vi "FlatToRichcif_channelcore_ForceChannel.vi"(5 "OutputClusterType":T1, 11 "InputCluster":T2) -> (3 "OutputCluster":T1)   [LabVIEW 2021, in "CIFCoreChannel_server.lvlib"]
uses:
  CIFCoreChannel_server.lvlib
  cif_channelcore_ForceChannel_Flat.ctl
  cif_channelcore_ForceChannel.ctl
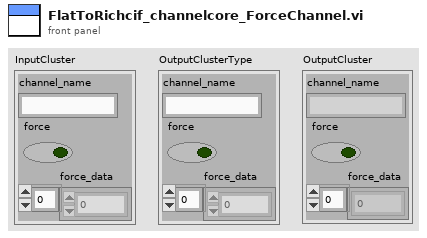
[diagram p1: front panel]
types:
  T1 = typedef "CIFCoreChannel_server.lvlib/cif_channelcore_ForceChannel.ctl" = cluster{"channel_name":string, "force":bool, "force_data":u8[]}
  T2 = typedef "CIFCoreChannel_server.lvlib/cif_channelcore_ForceChannel_Flat.ctl" = cluster{"channel_name":string, "force":bool, "force_data":u8[]}
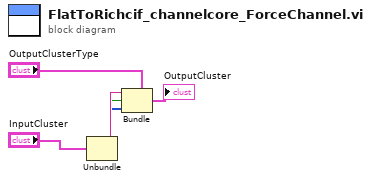
[diagram p0: block diagram]
diagram:
  n1 = Unbundle "Unbundle"("InputCluster") -> ("channel_name"=w3:string, "force"=w2:bool, "force_data"=w1:u8[])
  n2 = Bundle "Bundle"(cluster="OutputClusterType", "channel_name"=w3, "force"=w2, "force_data"=w1) -> (→"OutputCluster":T1)
